vi "Global.vi"() -> ()   [LabVIEW 2017]
panel:
  in  "Delta T":dbl=1.0
  in  "F-m'":dbl=1.0
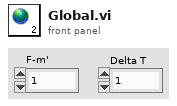
[diagram p1: front panel]
diagram:
